vi "rcs_cot.vi"(6 "range":dbl, 7 "Distance to RUT":dbl=3.0, 8 "Gain":dbl, 9 "GRX (dB)":dbl=10.0, 10 "GTX (dB)":dbl=10.0) -> (2 "x-y":dbl)   [LabVIEW 2015]
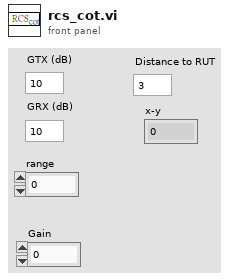
[diagram p1: front panel]
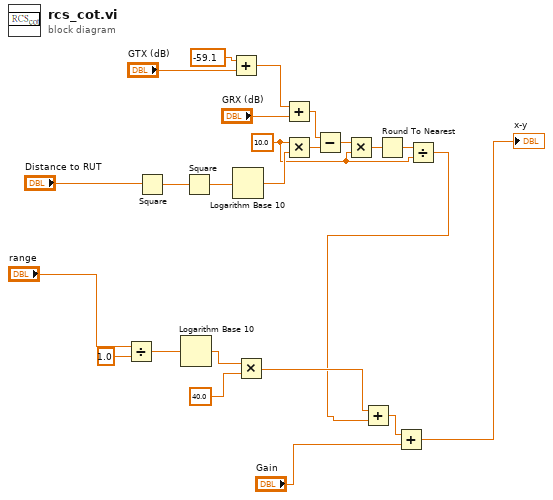
[diagram p0: block diagram]
diagram:
  w11 = 10.0 ("x")
  n1 = Divide(x="range", y=1.0) -> (x/y=w8:dbl)
  n2 = Square(x="Distance to RUT") -> (x^2=w19:dbl)
  n3 = Logarithm Base 10(1:w8) -> (0:w7:dbl)
  n4 = Square(x=w19) -> (x^2=w17:dbl)
  n5 = Add(x=-59.1, y="GTX (dB)") -> (x+y=w22:dbl)
  n6 = Logarithm Base 10(1:w17) -> (0:w16:dbl)
  n7 = Multiply(x=w7, y=40.0) -> (x*y=w5:dbl)
  n8 = Add(x=w22, y="GRX (dB)") -> (x+y=w18:dbl)
  n9 = Multiply(x=w11, y=w16) -> (x*y=w15:dbl)
  n10 = Subtract(x=w18, y=w15) -> (x-y=w14:dbl)
  n11 = Multiply(x=w14, y=w11) -> (x*y=w13:dbl)
  n12 = Round To Nearest(number=w13) -> (nearest integer value=w12:dbl)
  n13 = Divide(x=w12, y=w11) -> (x/y=w4:dbl)
  n14 = Add(x=w5, y=w4) -> (x+y=w3:dbl)
  n15 = Add(x=w3, y="Gain") -> (x+y=→"x-y":dbl)
